vi "HMF data.vi"(2 "DC offset":dbl, 3 "error in (no error)":errorcluster {"code" format="%.0x"}, 4 "VISA resource name":refnum<visa-resource-name>) -> (0 "error out":errorcluster {"code" format="%.0x"}, 1 "VISA resource name out":refnum<visa-resource-name>)   [LabVIEW 2015]
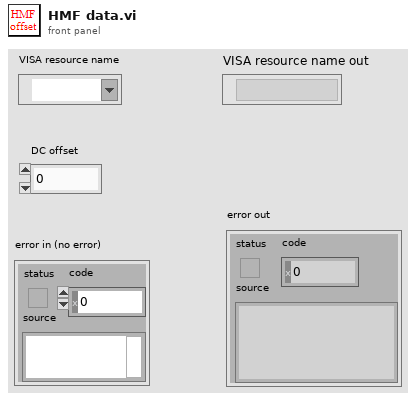
[diagram p1: front panel]
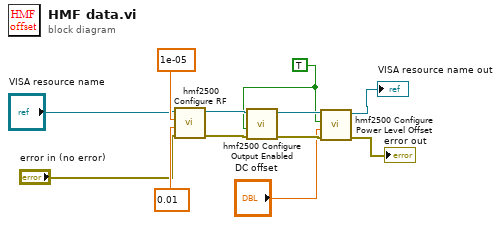
[diagram p0: block diagram]
diagram:
  w8 = TRUE
  n1 = call <instrlib>:"hmf2500 Configure RF.vi"("error in (no error)"="error in (no error)", "Power Level (0.2)"=0.01, "Frequency (1.0E6)"=1e-05, "VISA resource name"="VISA resource name") -> ("error out"=w11:errorcluster, "VISA resource name out"=w12:refnum<visa-resource-name>)  [unwired: 6 in]
  n2 = call <instrlib>:"hmf2500 Configure Output Enabled.vi"("error in (no error)"=w11, "Output Enabled (On)"=w8, "VISA resource name"=w12) -> ("error out"=w9:errorcluster, "VISA resource name out"=w10:refnum<visa-resource-name>)  [unwired: 7 in]
  n3 = call <instrlib>:"hmf2500 Configure Power Level Offset.vi"("error in (no error)"=w9, "Power Level Offset (5.0)"="DC offset", "Power Level (Off)"=w8, "VISA resource name"=w10) -> ("error out"=→"error out":errorcluster, "VISA resource name out"=→"VISA resource name out":refnum<visa-resource-name>)  [unwired: 6 in]
